vi "setRampParameters.vi"(8 "error in (no error)":errorcluster, 10 "RampParameters":T1, 11 "RampDown in":refnum<class "RampDown.lvclass">) -> (0 "error out":errorcluster, 3 "RampDown out":refnum<class "RampDown.lvclass">)   [LabVIEW 2011, in "Tools.lvlib" / "Scripting.lvlib" / "RampDown.lvclass"]
uses:
  RampDown.lvclass
  RampEvent/RampEvent.lvclass
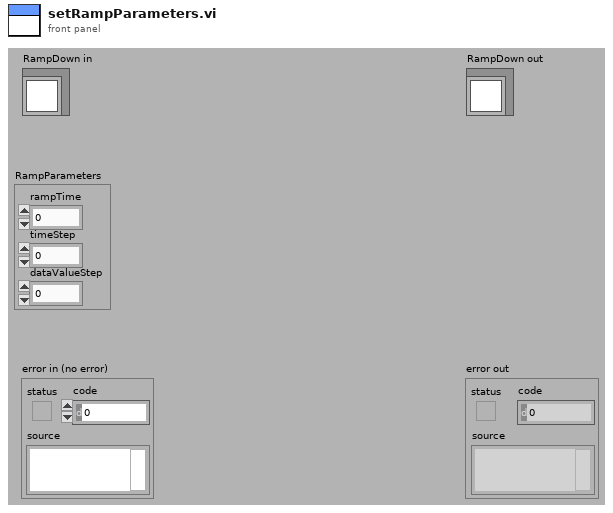
[diagram p1: front panel]
types:
  T1 = cluster{"rampTime":dbl, "timeStep":dbl, "dataValueStep":dbl}
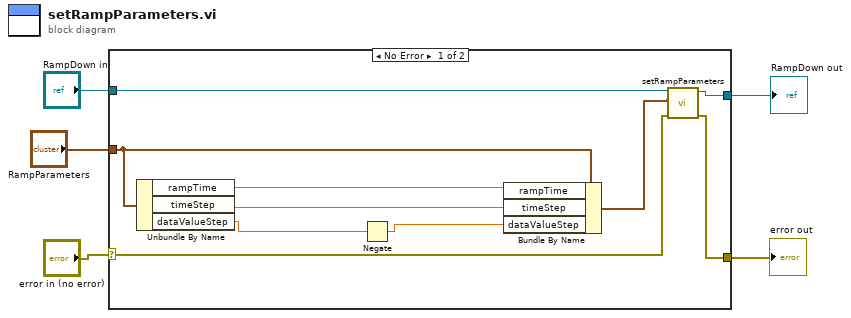
[diagram p0: block diagram]
diagram:
  n1 = case shown="No Error" "error in (no error)" {
    selector: "error in (no error)" -> [w8 w16]
    tunnel: "RampDown in" -> [w10 w17]
    tunnel: "RampParameters" -> [w15 _]
    tunnel: [w7 w16] -> w2
    tunnel: [w6 w17] -> w1
    frame No Error {
      n2 = Unbundle By Name(w15) -> ("rampTime"=w14:dbl, "timeStep"=w13:dbl, "dataValueStep"=w12:dbl)
      n3 = Negate(x=w12) -> (-x=w11:dbl)
      n4 = Bundle By Name(cluster=w15, "rampTime"=w14, "timeStep"=w13, "dataValueStep"=w11) -> (w9:T1)
      n5 = call-parent "setRampParameters.vi"("error in (no error)"=w8, "RampParameters"=w9, "RampEvent in"=w10) -> ("error out"=w7:errorcluster, "RampEvent out"=w6:refnum<class "RampDown.lvclass">)  [unwired: 7 in]
    }
    frame Error {
    }
  }
  "error out" <- w2
  "RampDown out" <- w1
